vi "SSC DCPower Configure Current Limit Array.vi"(0 "DCPower SSC in":T1[](array[typedef]), 5 "Current Limits (A)":dbl[](array[numeric]) format="%#_6p", 11 "error in":errorcluster) -> (4 "DCPower SSC out":T1[](array[typedef]), 15 "error out":errorcluster)   [LabVIEW 2020]
doc: "This VI configures the Current Limit.\n\nThis can be used when in the single point voltage mode."
uses:
  SSC DCPower.ctl
  0c094a83-1906-4472-bb05-463e0dd6146f.vi
  <vilib>/Utility/error.llb/Error Cluster From Error Code.vi
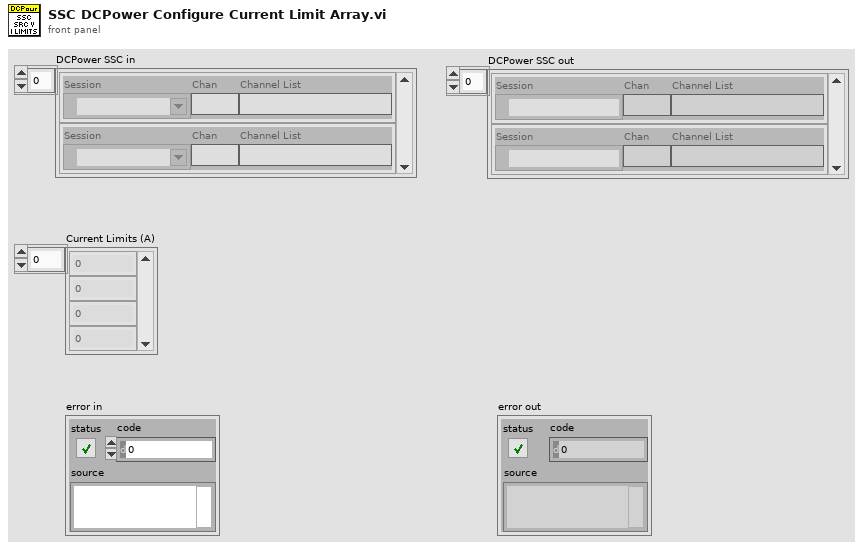
[diagram p1: front panel]
types:
  T1 = typedef "SSC DCPower.ctl" = cluster{"Session":refnum<k15>, "Chan":string, "Channel List":string}
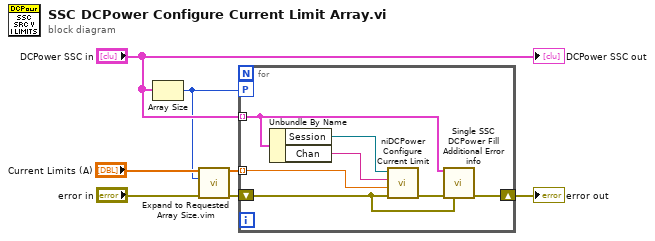
[diagram p0: block diagram]
diagram:
  n1 = Array Size(array="DCPower SSC in") -> (size(s)=w1:i32)
  n2 = call "Expand to Requested Array Size.vim"("Data In"="Current Limits (A)", "Requested Size"=w1, "error in"="error in") -> ("Data Out"=w2:dbl[], "error out"=w5:errorcluster)  [unwired: 11 in]
  n3 = for {
    tunnel: "DCPower SSC in" -> [w9] mode=indexing
    workers-P: w1 -> [_]
    tunnel: w2 -> [w13] mode=indexing
    shift-right: [w10] -> w7
    shift-left: w5 -> [w8]
    n4 = Unbundle By Name(w9) -> ("Session"=w12:refnum<k15>, "Chan"=w11:string)
    n5 = call <instrlib>:"niDCPower Configure Current Limit.vi"("error in (no error)"=w8, "current limit"=w13, "channel name"=w11, "instrument handle"=w12) -> ("error out"=w14:errorcluster)  [unwired: 6 in, 1 out]
    n6 = call "Single SSC DCPower Fill Additional Error info.vi"("DCPower SSC in"=w9, "error in"=w14, "previous error in"=w8) -> ("error out"=w10:errorcluster)  [unwired: 12 in]
  }
  "error out" <- w7
  "DCPower SSC out" <- "DCPower SSC in"
